vi "Reconfig Local Module.vi"(8 "error in (no error)":errorcluster, 9 "Config Channels":dbl[](array[numeric]), 10 "IOV ref":refnum<k21>, 11 "Module DVR":refnum<data-value>) -> (0 "error out":errorcluster)   [LabVIEW 2016, in "Scan Engine Custom Device.lvlib"]
uses:
  Scan Engine Custom Device.lvlib
  Modules.lvlibp/RSI Module/RSI Module.lvclass
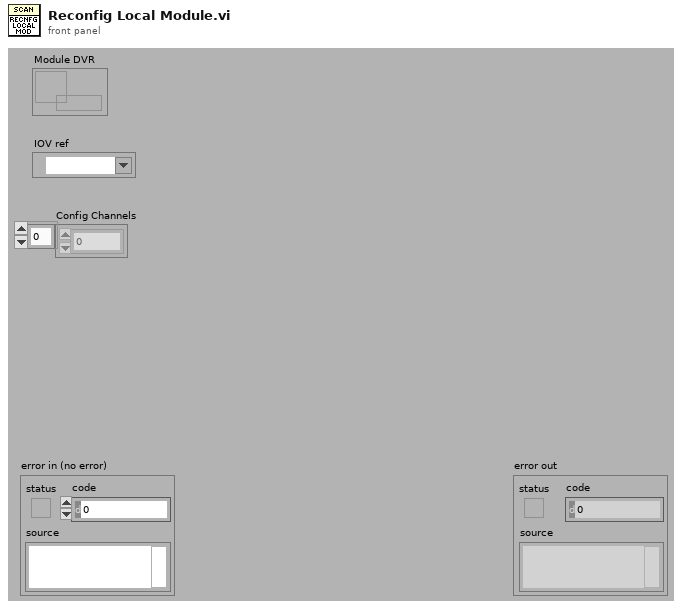
[diagram p1: front panel]
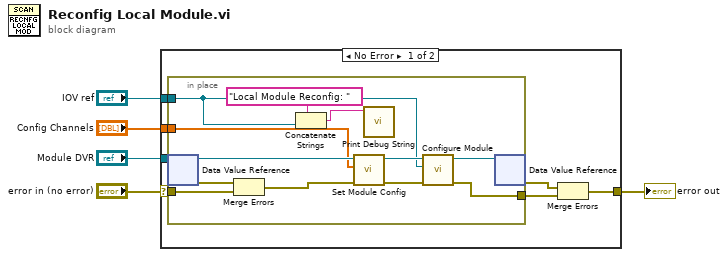
[diagram p0: block diagram]
diagram:
  n1 = case shown="No Error" "error in (no error)" {
    selector: "error in (no error)" -> [w11 w25]
    tunnel: [w6 w25] -> w4
    tunnel: "Module DVR" -> [w12 _]
    tunnel: "Config Channels" -> [w10 _]
    tunnel: "IOV ref" -> [w9 _]
    frame No Error {
      n2 = in-place {
        in-place-border: w11 -> [w23]
        in-place-border: w10 -> [w20]
        in-place-border: w9 -> [w13]
        in-place-border: [w16] -> w7
        n3 = in-place-dvr #1(w12) -> (w21:refnum<class "RSI Module.lvclass">, w24:errorcluster)
        n4 = Merge Errors(w24, w23) -> (w22:errorcluster)
        n5 = Concatenate Strings("Local Module Reconfig: " ("string"), w13) -> (w15:string)
        n6 = call-dynamic "Set Module Config.vi"("error in (no error)"=w22, "Config Channels"=w20, "RSI Module in"=w21) -> ("error out"=w19:errorcluster, "RSI Module out"=w18:refnum<class "RSI Module.lvclass">)  [unwired: 7 in]
        n7 = call "Print Debug String.vi"("String to write"=w15) -> ()  [unwired: 9 in, 1 out]
        n8 = call-dynamic "Configure Module.vi"("error in (no error)"=w19, "IOV ref in"=w13, "RSI Module in"=w18) -> ("error out"=w16:errorcluster, "RSI Module out"=w17:refnum<class "RSI Module.lvclass">)  [unwired: 6 in, 1 out]
        n9 = in-place-dvr #1(w17) -> (w8:errorcluster)  [unwired: 1 out]
      }
      n10 = Merge Errors(w8, w7) -> (w6:errorcluster)
    }
    frame Error {
    }
  }
  "error out" <- w4
